vi "TCP-IP Q_Bridge.Rcv Check VerifyHandShake.vi"(10 "Msg In":string, 11 "ConID":refnum<k5>) -> (2 "Msg Out":string, 3 "ConID Out":refnum<k5>, 5 "Is Ver":bool)   [LabVIEW 2018, in "KATE_Lib.lvlib" / "TCP-IP.lvlib"]
uses:
  TCP-IP.lvlib
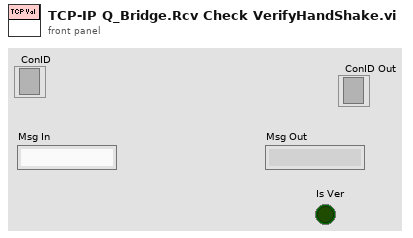
[diagram p1: front panel]
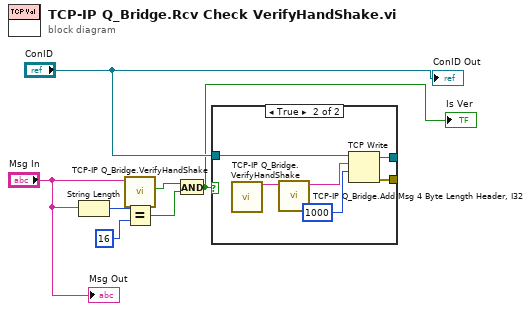
[diagram p0: block diagram]
diagram:
  n1 = String Length(string="Msg In") -> (length=w6:i32)
  n2 = call "TCP-IP Q_Bridge.VerifyHandShake.vi"("Msg In"="Msg In") -> ("OK"=w4:bool)  [unwired: 9 in, 1 out]
  n3 = Equal?(x=w6, y=16) -> (x = y?=w3:bool)
  n4 = And(x=w4, y=w3) -> (x .and. y?=w1:bool)
  "Is Ver" <- w1
  n5 = case shown="True" w1 {
    tunnel: [_ w12] -> _
    tunnel: [_ w11] -> _
    tunnel: "ConID" -> [_ w8]
    frame False {
    }
    frame True {
      n6 = call "TCP-IP Q_Bridge.VerifyHandShake.vi"() -> ("Msg Out"=w9:string)  [unwired: 10 in, 1 out]
      n7 = call "TCP-IP Q_Bridge.Add Msg 4 Byte Length Header, I32.vi"("Message"=w9) -> ("Message + Header"=w13:string)  [unwired: 10 in]
      n8 = TCP Write(connection ID=w8, data in=w13, 9:1000 ("timeout ms (25000)")) -> (connection ID out=w12:refnum<k5>, error out=w11:errorcluster)  [unwired: 1 in, 1 out]
    }
  }
  "ConID Out" <- "ConID"
  "Msg Out" <- "Msg In"
